vi "RubikTurnFSM(obsolet).vi"() -> ()   [LabVIEW 2017]
doc: "The myRIO Project template acquires acceleration data from the onboard accelerometer and displays the changes of acceleration values in a waveform chart."
uses:
  Projekt-RubikLibrary/ServoEnumControl.ctl
  Projekt-RubikLibrary/ServoAbsAngleControl_.ctl
  Projekt-RubikLibrary/RubikLibrary.lvlib
panel:
  in  "Turn by":enum16{"-90°", "+90°"}(ring)
  in  "Servo":T1
  out "error out":errorcluster
  # "Overview:  A finite state machine so that we can use our servos to turn the cube's faces multiple times, back and forth.\nInstructions:\n1. Check the myRIO target IP address in the project and make sure the target IP address is correct. \n2. Run this VI."
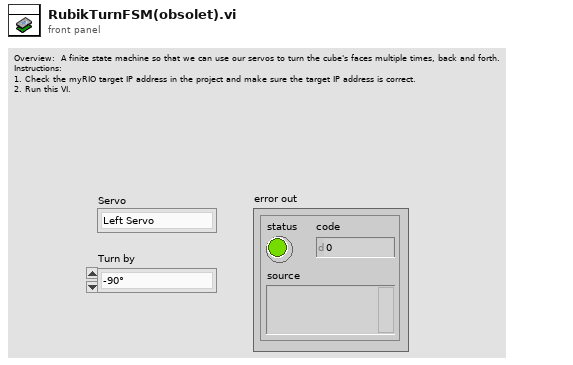
[diagram p1: front panel]
types:
  T1 = typedef "RubikLibrary.lvlib/ServoEnumControl.ctl" = enum16{"Left Servo", "Front Servo", "Right Servo"}
  T2 = typedef "ServoAbsAngleControl_.ctl" = enum16{"-90°", "0°", "+90°"}
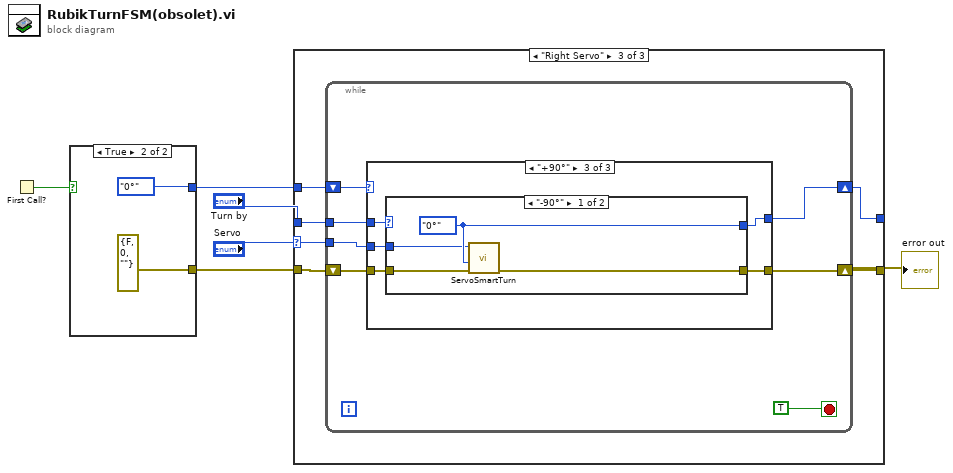
[diagram p0: block diagram]
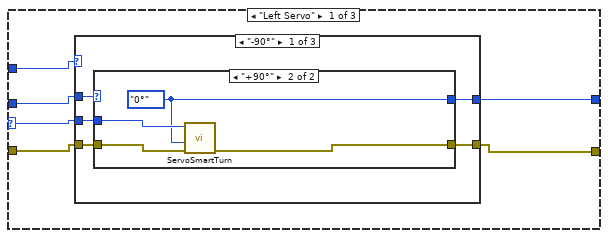
[diagram p2: hidden frame]
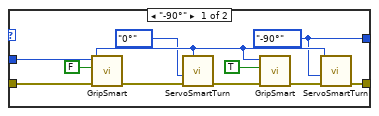
[diagram p3: hidden frame]
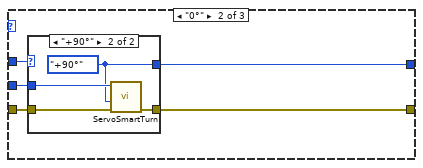
[diagram p4: hidden frame]
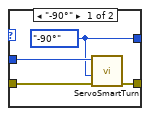
[diagram p5: hidden frame]
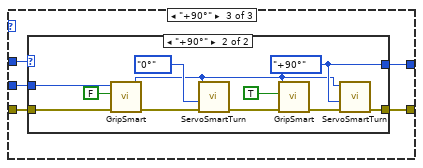
[diagram p6: hidden frame]
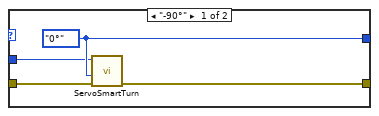
[diagram p7: hidden frame]
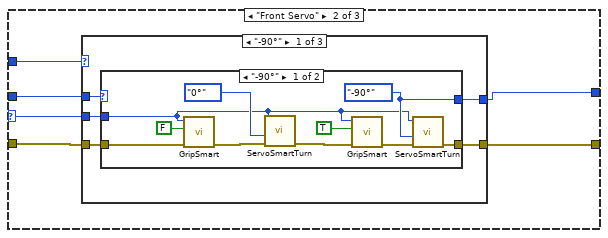
[diagram p8: hidden frame]
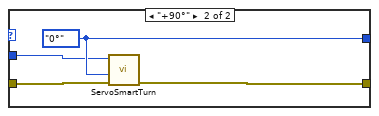
[diagram p9: hidden frame]
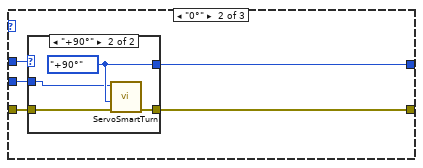
[diagram p10: hidden frame]
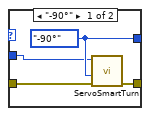
[diagram p11: hidden frame]
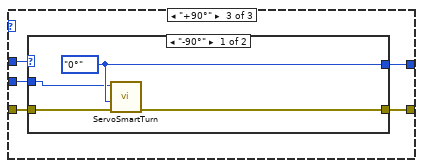
[diagram p12: hidden frame]
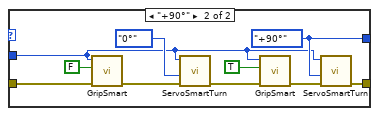
[diagram p13: hidden frame]
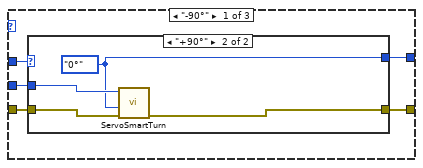
[diagram p14: hidden frame]
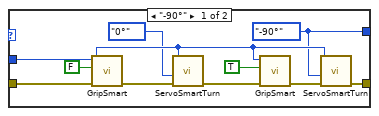
[diagram p15: hidden frame]
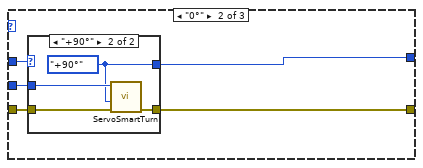
[diagram p16: hidden frame]
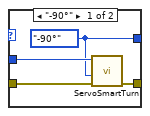
[diagram p17: hidden frame]
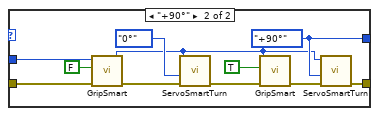
[diagram p18: hidden frame]
diagram:
  n1 = First Call?() -> (First Call?: T/F=w3:bool)
  n2 = case shown="True" w3 {
    tunnel: [_ errorcluster {"status"=FALSE, "code"=0, "source"=""} ("error in (no error)")] -> w6
    tunnel: [_ ServoAbsAngleControl_."0°" ("Turn to")] -> w5
    frame False {
    }
    frame True {
    }
  }
  n3 = case shown="\"Right Servo\"" "Servo" {
    selector: "Servo" -> [w12 w69 w126]
    tunnel: [w14 w67 w124] -> _
    tunnel: "Turn by" -> [w13 w70 w127]
    tunnel: w5 -> [w11 w71 w128]
    tunnel: w6 -> [w10 w68 w125]
    tunnel: [w9 w66 w123] -> w4
    frame "Left Servo" {
      n4 = case shown="\"-90°\"" w11 {
        tunnel: w13 -> [w18 w38 w51]
        tunnel: [w19 w37 w50] -> w14
        tunnel: w12 -> [w17 w36 w49]
        tunnel: w10 -> [w16 w35 w48]
        tunnel: [w15 w34 w47] -> w9
        frame "-90°" {
          n5 = case shown="\"+90°\"" w18 {
            tunnel: [w22 w32] -> w19
            tunnel: w17 -> [w26 w33]
            tunnel: w16 -> [w21 w31]
            tunnel: [w20 w30] -> w15
            frame "-90°" {
              w22 = ServoAbsAngleControl_."-90°" ("Turn to")
              n6 = call "GripSmart.vi"("error in"=w21, "Turn to (in)"=FALSE, "Servo"=w26) -> ("error out"=w29:errorcluster)  [unwired: 7 in, 1 out]
              n7 = call "ServoSmartTurn.vi"("error in"=w29, "Turn to (in)"=ServoAbsAngleControl_."0°", "Servo"=w26) -> ("error out"=w28:errorcluster)  [unwired: 7 in, 1 out]
              n8 = call "GripSmart.vi"("error in"=w28, "Turn to (in)"=TRUE, "Servo"=w26) -> ("error out"=w27:errorcluster)  [unwired: 7 in, 1 out]
              n9 = call "ServoSmartTurn.vi"("error in"=w27, "Turn to (in)"=w22, "Servo"=w26) -> ("error out"=w20:errorcluster)  [unwired: 7 in, 1 out]
            }
            frame "+90°" {
              w32 = ServoAbsAngleControl_."0°" ("Turn to")
              n10 = call "ServoSmartTurn.vi"("error in"=w31, "Turn to (in)"=w32, "Servo"=w33) -> ("error out"=w30:errorcluster)  [unwired: 7 in, 1 out]
            }
          }
        }
        frame "0°" {
          n11 = case shown="\"+90°\"" w38 {
            tunnel: [w41 w45] -> w37
            tunnel: w36 -> [w42 w46]
            tunnel: w35 -> [w39 w43]
            tunnel: [w40 w44] -> w34
            frame "-90°" {
              w41 = ServoAbsAngleControl_."-90°" ("Turn to")
              n12 = call "ServoSmartTurn.vi"("error in"=w39, "Turn to (in)"=w41, "Servo"=w42) -> ("error out"=w40:errorcluster)  [unwired: 7 in, 1 out]
            }
            frame "+90°" {
              w45 = ServoAbsAngleControl_."+90°" ("Turn to")
              n13 = call "ServoSmartTurn.vi"("error in"=w43, "Turn to (in)"=w45, "Servo"=w46) -> ("error out"=w44:errorcluster)  [unwired: 7 in, 1 out]
            }
          }
        }
        frame "+90°" {
          n14 = case shown="\"+90°\"" w51 {
            tunnel: [w55 w59] -> w50
            tunnel: w49 -> [w54 w56]
            tunnel: w48 -> [w53 w58]
            tunnel: [w52 w57] -> w47
            frame "-90°" {
              w55 = ServoAbsAngleControl_."0°" ("Turn to")
              n15 = call "ServoSmartTurn.vi"("error in"=w53, "Turn to (in)"=w55, "Servo"=w54) -> ("error out"=w52:errorcluster)  [unwired: 7 in, 1 out]
            }
            frame "+90°" {
              w59 = ServoAbsAngleControl_."+90°" ("Turn to")
              n16 = call "GripSmart.vi"("error in"=w58, "Turn to (in)"=FALSE, "Servo"=w56) -> ("error out"=w65:errorcluster)  [unwired: 7 in, 1 out]
              n17 = call "ServoSmartTurn.vi"("error in"=w65, "Turn to (in)"=ServoAbsAngleControl_."0°", "Servo"=w56) -> ("error out"=w64:errorcluster)  [unwired: 7 in, 1 out]
              n18 = call "GripSmart.vi"("error in"=w64, "Turn to (in)"=TRUE, "Servo"=w56) -> ("error out"=w63:errorcluster)  [unwired: 7 in, 1 out]
              n19 = call "ServoSmartTurn.vi"("error in"=w63, "Turn to (in)"=w59, "Servo"=w56) -> ("error out"=w57:errorcluster)  [unwired: 7 in, 1 out]
            }
          }
        }
      }
    }
    frame "Front Servo" {
      n20 = case shown="\"-90°\"" w71 {
        tunnel: [w76 w95 w108] -> w67
        tunnel: [w75 w94 w107] -> w66
        tunnel: w70 -> [w74 w93 w105]
        tunnel: w69 -> [w73 w92 w106]
        tunnel: w68 -> [w72 w91 w104]
        frame "-90°" {
          n21 = case shown="\"-90°\"" w74 {
            tunnel: [w80 w90] -> w76
            tunnel: [w79 w89] -> w75
            tunnel: w73 -> [w77 w88]
            tunnel: w72 -> [w78 w87]
            frame "-90°" {
              w80 = ServoAbsAngleControl_."-90°" ("Turn to")
              n22 = call "GripSmart.vi"("error in"=w78, "Turn to (in)"=FALSE, "Servo"=w77) -> ("error out"=w86:errorcluster)  [unwired: 7 in, 1 out]
              n23 = call "ServoSmartTurn.vi"("error in"=w86, "Turn to (in)"=ServoAbsAngleControl_."0°", "Servo"=w77) -> ("error out"=w85:errorcluster)  [unwired: 7 in, 1 out]
              n24 = call "GripSmart.vi"("error in"=w85, "Turn to (in)"=TRUE, "Servo"=w77) -> ("error out"=w84:errorcluster)  [unwired: 7 in, 1 out]
              n25 = call "ServoSmartTurn.vi"("error in"=w84, "Turn to (in)"=w80, "Servo"=w77) -> ("error out"=w79:errorcluster)  [unwired: 7 in, 1 out]
            }
            frame "+90°" {
              w90 = ServoAbsAngleControl_."0°" ("Turn to")
              n26 = call "ServoSmartTurn.vi"("error in"=w87, "Turn to (in)"=w90, "Servo"=w88) -> ("error out"=w89:errorcluster)  [unwired: 7 in, 1 out]
            }
          }
        }
        frame "0°" {
          n27 = case shown="\"+90°\"" w93 {
            tunnel: [w99 w103] -> w95
            tunnel: [w98 w102] -> w94
            tunnel: w92 -> [w97 w101]
            tunnel: w91 -> [w96 w100]
            frame "-90°" {
              w99 = ServoAbsAngleControl_."-90°" ("Turn to")
              n28 = call "ServoSmartTurn.vi"("error in"=w96, "Turn to (in)"=w99, "Servo"=w97) -> ("error out"=w98:errorcluster)  [unwired: 7 in, 1 out]
            }
            frame "+90°" {
              w103 = ServoAbsAngleControl_."+90°" ("Turn to")
              n29 = call "ServoSmartTurn.vi"("error in"=w100, "Turn to (in)"=w103, "Servo"=w101) -> ("error out"=w102:errorcluster)  [unwired: 7 in, 1 out]
            }
          }
        }
        frame "+90°" {
          n30 = case shown="\"-90°\"" w105 {
            tunnel: [w112 w116] -> w108
            tunnel: [w111 w115] -> w107
            tunnel: w106 -> [w110 w114]
            tunnel: w104 -> [w109 w113]
            frame "-90°" {
              w112 = ServoAbsAngleControl_."0°" ("Turn to")
              n31 = call "ServoSmartTurn.vi"("error in"=w109, "Turn to (in)"=w112, "Servo"=w110) -> ("error out"=w111:errorcluster)  [unwired: 7 in, 1 out]
            }
            frame "+90°" {
              w116 = ServoAbsAngleControl_."+90°" ("Turn to")
              n32 = call "GripSmart.vi"("error in"=w113, "Turn to (in)"=FALSE, "Servo"=w114) -> ("error out"=w122:errorcluster)  [unwired: 7 in, 1 out]
              n33 = call "ServoSmartTurn.vi"("error in"=w122, "Turn to (in)"=ServoAbsAngleControl_."0°", "Servo"=w114) -> ("error out"=w121:errorcluster)  [unwired: 7 in, 1 out]
              n34 = call "GripSmart.vi"("error in"=w121, "Turn to (in)"=TRUE, "Servo"=w114) -> ("error out"=w120:errorcluster)  [unwired: 7 in, 1 out]
              n35 = call "ServoSmartTurn.vi"("error in"=w120, "Turn to (in)"=w116, "Servo"=w114) -> ("error out"=w115:errorcluster)  [unwired: 7 in, 1 out]
            }
          }
        }
      }
    }
    frame "Right Servo" {
      n36 = while {
        tunnel: w127 -> [w134]
        tunnel: w126 -> [w133]
        shift-right: [w131] -> w124
        shift-left: w128 -> [w135]
        shift-right: [w130] -> w123
        shift-left: w125 -> [w132]
        stop <- TRUE stop-if-true
        n37 = case shown="\"+90°\"" w135 {
          tunnel: [w140 w159 w172] -> w131
          tunnel: w133 -> [w139 w158 w171]
          tunnel: w132 -> [w138 w157 w170]
          tunnel: [w137 w156 w169] -> w130
          tunnel: w134 -> [w136 w155 w168]
          frame "-90°" {
            n38 = case shown="\"+90°\"" w136 {
              tunnel: [w143 w153] -> w140
              tunnel: w139 -> [w147 w154]
              tunnel: w138 -> [w142 w152]
              tunnel: [w141 w151] -> w137
              frame "-90°" {
                w143 = ServoAbsAngleControl_."-90°" ("Turn to")
                n39 = call "GripSmart.vi"("error in"=w142, "Turn to (in)"=FALSE, "Servo"=w147) -> ("error out"=w150:errorcluster)  [unwired: 7 in, 1 out]
                n40 = call "ServoSmartTurn.vi"("error in"=w150, "Turn to (in)"=ServoAbsAngleControl_."0°", "Servo"=w147) -> ("error out"=w149:errorcluster)  [unwired: 7 in, 1 out]
                n41 = call "GripSmart.vi"("error in"=w149, "Turn to (in)"=TRUE, "Servo"=w147) -> ("error out"=w148:errorcluster)  [unwired: 7 in, 1 out]
                n42 = call "ServoSmartTurn.vi"("error in"=w148, "Turn to (in)"=w143, "Servo"=w147) -> ("error out"=w141:errorcluster)  [unwired: 7 in, 1 out]
              }
              frame "+90°" {
                w153 = ServoAbsAngleControl_."0°" ("Turn to")
                n43 = call "ServoSmartTurn.vi"("error in"=w152, "Turn to (in)"=w153, "Servo"=w154) -> ("error out"=w151:errorcluster)  [unwired: 7 in, 1 out]
              }
            }
          }
          frame "0°" {
            n44 = case shown="\"+90°\"" w155 {
              tunnel: [w162 w166] -> w159
              tunnel: w158 -> [w163 w167]
              tunnel: w157 -> [w160 w164]
              tunnel: [w161 w165] -> w156
              frame "-90°" {
                w162 = ServoAbsAngleControl_."-90°" ("Turn to")
                n45 = call "ServoSmartTurn.vi"("error in"=w160, "Turn to (in)"=w162, "Servo"=w163) -> ("error out"=w161:errorcluster)  [unwired: 7 in, 1 out]
              }
              frame "+90°" {
                w166 = ServoAbsAngleControl_."+90°" ("Turn to")
                n46 = call "ServoSmartTurn.vi"("error in"=w164, "Turn to (in)"=w166, "Servo"=w167) -> ("error out"=w165:errorcluster)  [unwired: 7 in, 1 out]
              }
            }
          }
          frame "+90°" {
            n47 = case shown="\"-90°\"" w168 {
              tunnel: [w176 w180] -> w172
              tunnel: w171 -> [w175 w177]
              tunnel: w170 -> [w174 w179]
              tunnel: [w173 w178] -> w169
              frame "-90°" {
                w176 = ServoAbsAngleControl_."0°" ("Turn to")
                n48 = call "ServoSmartTurn.vi"("error in"=w174, "Turn to (in)"=w176, "Servo"=w175) -> ("error out"=w173:errorcluster)  [unwired: 7 in, 1 out]
              }
              frame "+90°" {
                w180 = ServoAbsAngleControl_."+90°" ("Turn to")
                n49 = call "GripSmart.vi"("error in"=w179, "Turn to (in)"=FALSE, "Servo"=w177) -> ("error out"=w186:errorcluster)  [unwired: 7 in, 1 out]
                n50 = call "ServoSmartTurn.vi"("error in"=w186, "Turn to (in)"=ServoAbsAngleControl_."0°", "Servo"=w177) -> ("error out"=w185:errorcluster)  [unwired: 7 in, 1 out]
                n51 = call "GripSmart.vi"("error in"=w185, "Turn to (in)"=TRUE, "Servo"=w177) -> ("error out"=w184:errorcluster)  [unwired: 7 in, 1 out]
                n52 = call "ServoSmartTurn.vi"("error in"=w184, "Turn to (in)"=w180, "Servo"=w177) -> ("error out"=w178:errorcluster)  [unwired: 7 in, 1 out]
              }
            }
          }
        }
      }
    }
  }
  "error out" <- w4
